vi "ppm err.vi"(1 "Actual":dbl, 2 "Expected":dbl) -> (0 "Err (ppm)":dbl)   [LabVIEW 2010]
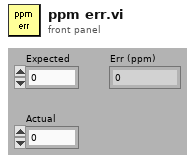
[diagram p1: front panel]
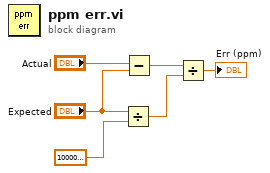
[diagram p0: block diagram]
diagram:
  n1 = Divide(x="Expected", y=1000000.0) -> (x/y=w2:dbl)
  n2 = Subtract(x="Actual", y="Expected") -> (x-y=w5:dbl)
  n3 = Divide(x=w5, y=w2) -> (x/y=→"Err (ppm)":dbl)
